vi "init.vi"(0 "ConfigureILCGPIStrategy in":refnum<class "ConfigureILCGPIStrategy.lvclass">, 1 "MUX Settings":T3, 2 "MUX Signals":T1, 3 "DAQ Channel To Write":refnum<k21>, 4 "Digital Signal Level":T2, 5 "error in (no error)":errorcluster) -> (14 "ConfigureILCGPIStrategy out":refnum<class "ConfigureILCGPIStrategy.lvclass">, 19 "error out":errorcluster)   [LabVIEW 2015, in "ConfigureILCGPIStrategy.lvclass"]
uses:
  ConfigureILCGPIStrategy.lvclass
  Typedefs/MUX Settings.ctl
  Typedefs/Digital Signal Level.ctl
  Typedefs/MUX Signals.ctl
  ConfigureILCGPIStrategy.lvclass/ConfigureILCGPIStrategy.ctl
  Typedefs/ILCBTTypedefs.lvlib
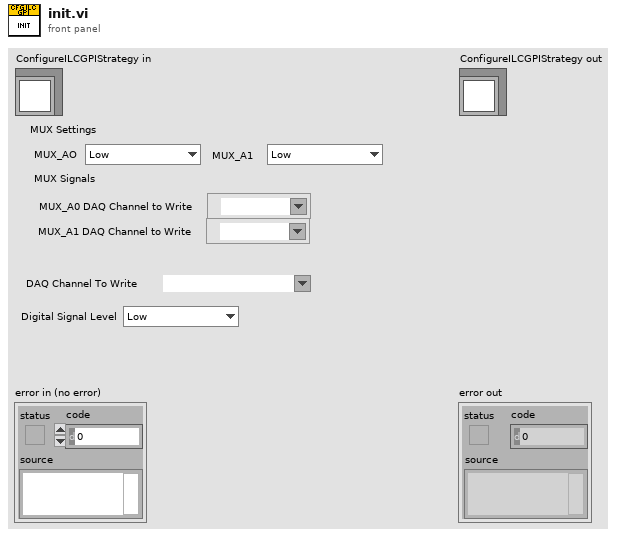
[diagram p1: front panel]
types:
  T1 = typedef "ILCBTTypedefs.lvlib/MUX Signals.ctl" = cluster{"MUX_A0 DAQ Channel to Write":refnum<k21>, "MUX_A1 DAQ Channel to Write":refnum<k21>}
  T2 = typedef "ILCBTTypedefs.lvlib/Digital Signal Level.ctl" = enum16{"Low", "High"}
  T3 = typedef "ILCBTTypedefs.lvlib/MUX Settings.ctl" = cluster{"MUX_AO":T2, "MUX_A1":T2}
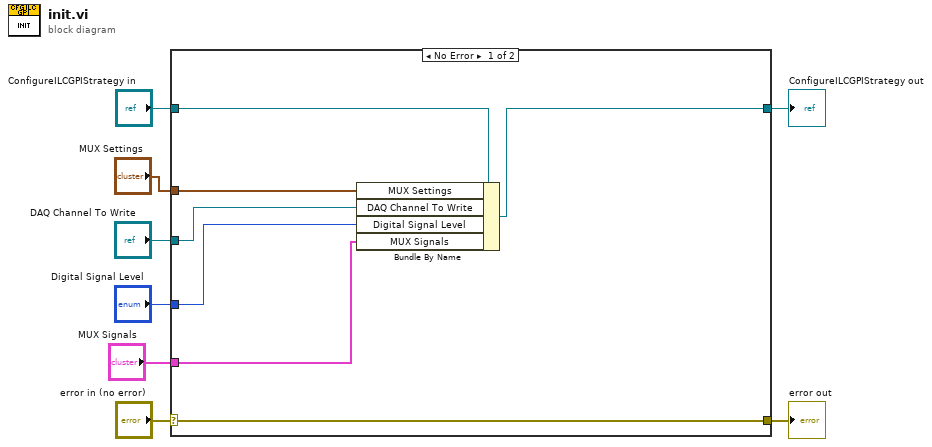
[diagram p0: block diagram]
diagram:
  n1 = case shown="No Error" "error in (no error)" {
    selector: "error in (no error)" -> [w15 w17]
    tunnel: [w15 w17] -> w7
    tunnel: [w13 w16] -> w5
    tunnel: "ConfigureILCGPIStrategy in" -> [w14 w16]
    tunnel: "MUX Settings" -> [w12 _]
    tunnel: "DAQ Channel To Write" -> [w11 _]
    tunnel: "Digital Signal Level" -> [w10 _]
    tunnel: "MUX Signals" -> [w9 _]
    frame No Error {
      n2 = Bundle By Name(cluster=w14, "MUX Settings"=w12, "DAQ Channel To Write"=w11, "Digital Signal Level"=w10, "MUX Signals"=w9) -> (w13:refnum<class "ConfigureILCGPIStrategy.lvclass">)
    }
    frame Error {
    }
  }
  "error out" <- w7
  "ConfigureILCGPIStrategy out" <- w5
